vi "Search.vi"(8 "error in (no error)":errorcluster, 11 "LinkedList in":refnum<class "LinkedList.lvclass">) -> (0 "error out":errorcluster, 1 "found":bool, 2 "Node":refnum<data-value>, 3 "LinkedList out":refnum<class "LinkedList.lvclass">)   [LabVIEW 2013, in "LinkedList.lvclass"]
doc: "Searches a linked list and returns the node if found. You must override IsSearchGoalNode.vi to determine the goal node of the search."
uses:
  LinkedList.lvclass
  LLNode/LLNode.lvclass
  LinkedList.lvclass/LinkedList.ctl
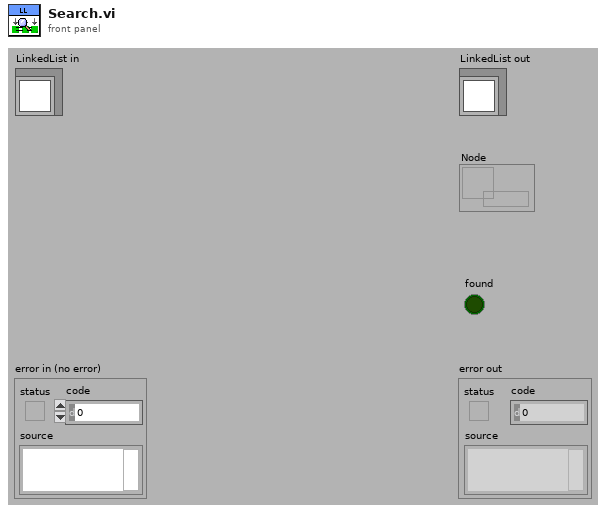
[diagram p1: front panel]
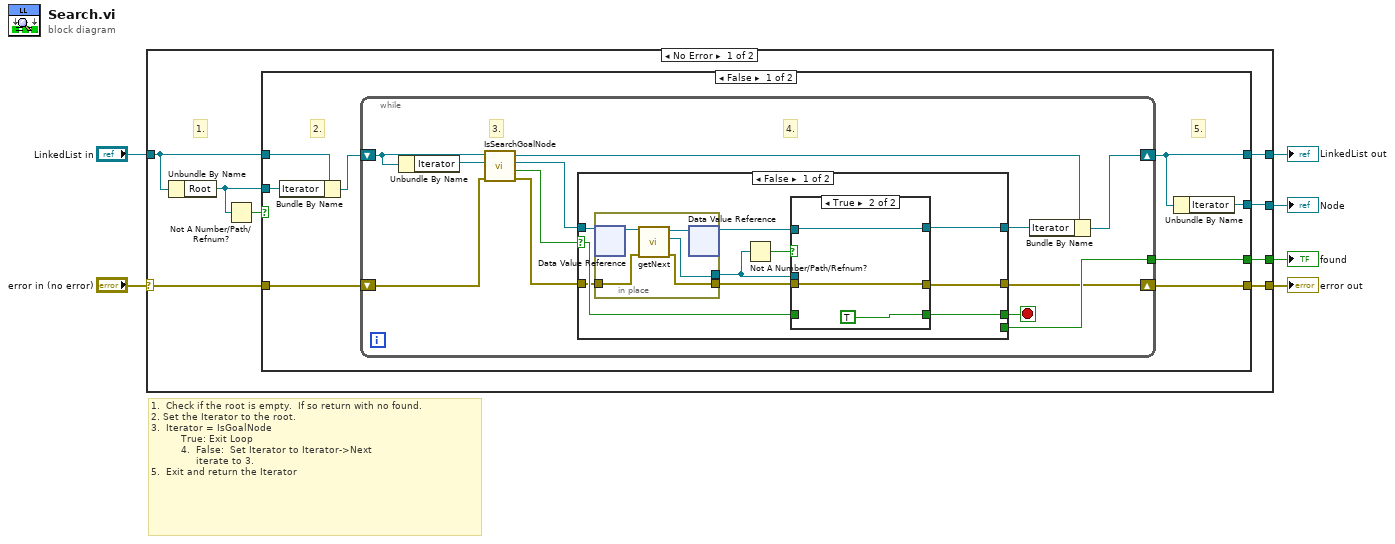
[diagram p0: block diagram]
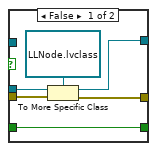
[diagram p2: hidden frame]
diagram:
  # "1.  Check if the root is empty.  If so return with no found.\n2. Set the Iterator to the root.\n3.  Iterator = IsGoalNode\n          True: Exit Loop \n          4.  False:  Set Iterator to Iterator->Next\n               iterate to 3.\n5.  Exit and return the Iterator"
  n1 = case shown="No Error" "error in (no error)" {
    selector: "error in (no error)" -> [w10 w65]
    tunnel: [w9 w65] -> w5
    tunnel: [w12 w64] -> w3
    tunnel: "LinkedList in" -> [w14 w64]
    tunnel: [w13 _] -> w2
    tunnel: [w11 _] -> w1
    frame No Error {
      # "1."
      n2 = Unbundle By Name(w14) -> ("Root"=w8:refnum<data-value>)
      n3 = Not A Number/Path/Refnum?(number/path/refnum=w8) -> (NaN/Path/Refnum?=w7:bool)
      n4 = case shown="False" w7 {
        tunnel: w14 -> [w22 w63]
        tunnel: [w20 _] -> w13
        tunnel: [w19 w63] -> w12
        tunnel: [w18 _] -> w11
        tunnel: w10 -> [w17 w62]
        tunnel: [w16 w62] -> w9
        tunnel: w8 -> [w15 _]
        frame False {
          # "5."
          # "2."
          n5 = Bundle By Name(cluster=w22, "Iterator"=w15) -> (w21:refnum<class "LinkedList.lvclass">)
          n6 = while {
            shift-right: [w34] -> w19
            shift-left: w21 -> [w29]
            tunnel: [w32] -> w18
            shift-right: [w31] -> w16
            shift-left: w17 -> [w25]
            stop <- w33 stop-if-true
            # "4."
            # "3."
            n7 = Unbundle By Name(w29) -> ("Iterator"=w27:refnum<data-value>)
            n8 = call-dynamic "IsSearchGoalNode.vi"("error in (no error)"=w25, "NodeToIdentify in"=w27, "LinkedList in"=w29) -> ("error out"=w24:errorcluster, "IsGoalNode"=w23:bool, "NodeToIdentify out"=w26:refnum<data-value>, "LinkedList out"=w28:refnum<class "LinkedList.lvclass">)  [unwired: 5 in]
            n9 = case shown="False" w23 {
              selector: w23 -> [w42 w60]
              tunnel: [w40 w60] -> w33
              tunnel: [w43 w61] -> w30
              tunnel: w26 -> [w44 w61]
              tunnel: [_ w60] -> w32
              tunnel: w24 -> [w37 w59]
              tunnel: [w35 w59] -> w31
              frame False {
                n10 = in-place {
                  in-place-border: [w56] -> w39
                  in-place-border: w37 -> [w55]
                  in-place-border: [w54] -> w36
                  n11 = in-place-dvr #1(w44) -> (w58:refnum<class "LLNode.lvclass">)  [unwired: 1 out]
                  n12 = call "getNext.vi"("error in (no error)"=w55, "LLNode in"=w58) -> ("error out"=w54:errorcluster, "next"=w56:refnum<data-value>, "LLNode out"=w57:refnum<class "LLNode.lvclass">)  [unwired: 7 in]
                  n13 = in-place-dvr #1(w57) -> (w38:refnum<data-value>)  [unwired: 1 out]
                }
                n14 = Not A Number/Path/Refnum?(number/path/refnum=w39) -> (NaN/Path/Refnum?=w41:bool)
                n15 = case shown="True" w41 {
                  tunnel: [w49 w52] -> w43
                  tunnel: w39 -> [w48 _]
                  tunnel: w42 -> [w47 _]
                  tunnel: [w47 TRUE] -> w40
                  tunnel: w38 -> [_ w52]
                  tunnel: w36 -> [w46 w51]
                  tunnel: [w45 w51] -> w35
                  frame False {
                    n16 = To More Specific Class(target class=refnum<data-value> refnum ("Iterator"), reference=w48, error in=w46) -> (specific class reference=w49:refnum<data-value>, error out=w45:errorcluster)
                  }
                  frame True {
                  }
                }
              }
              frame True {
              }
            }
            n17 = Bundle By Name(cluster=w28, "Iterator"=w30) -> (w34:refnum<class "LinkedList.lvclass">)
          }
          n18 = Unbundle By Name(w19) -> ("Iterator"=w20:refnum<data-value>)
        }
        frame True {
        }
      }
    }
    frame Error {
    }
  }
  "error out" <- w5
  "LinkedList out" <- w3
  "Node" <- w2
  "found" <- w1
